vi "Write Analogue.vi"(8 "error in (no error)":errorcluster, 9 "Output":bool, 10 "Channel index(0)":i32, 11 "Lambda Gen Plus in":refnum<class "Lambda Gen Plus.lvclass">) -> (0 "error out":errorcluster, 2 "Success?":bool, 3 "Lambda Gen Plus out":refnum<class "Lambda Gen Plus.lvclass">)   [LabVIEW 2025, in "Power Supply.lvlib" / "Lambda Gen Plus.lvclass"]
uses:
  Lambda Gen Plus.lvclass
  Lambda Gen Plus.lvclass/Lambda Gen Plus.ctl
  <instrlib>/TDK-Lambda G Series/TDK-Lambda G Series.lvlib
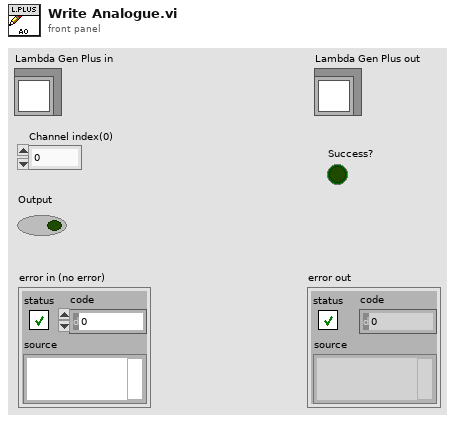
[diagram p1: front panel]
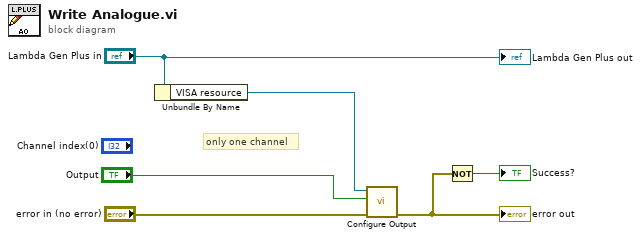
[diagram p0: block diagram]
diagram:
  # "only one channel"
  n1 = Unbundle By Name("Lambda Gen Plus in") -> ("VISA resource"=w4:refnum<visa-resource-name>)
  n2 = call <instrlib>:"Configure Output.vi"("error in (no error)"="error in (no error)", "Enable Output (False)"="Output", "VISA resource name"=w4) -> ("error out"=w2:errorcluster)  [unwired: 7 in, 1 out]
  "error out" <- w2
  n3 = Not(x=w2) -> (.not. x?=→"Success?":bool)
  "Lambda Gen Plus out" <- "Lambda Gen Plus in"
